vi "GetChildByName.vi"(8 "error in (no error)":errorcluster, 10 "BrowerComponentID(\"\")":string, 11 "reference in":refnum<class "BrowerComponent.lvclass">) -> (0 "error out":errorcluster, 2 "BrowerComponent":refnum<class "BrowerComponent.lvclass">, 3 "reference out":refnum<class "BrowerComponent.lvclass">)   [LabVIEW 2015, in "BrowerComponent.lvclass"]
uses:
  BrowerComponent.lvclass
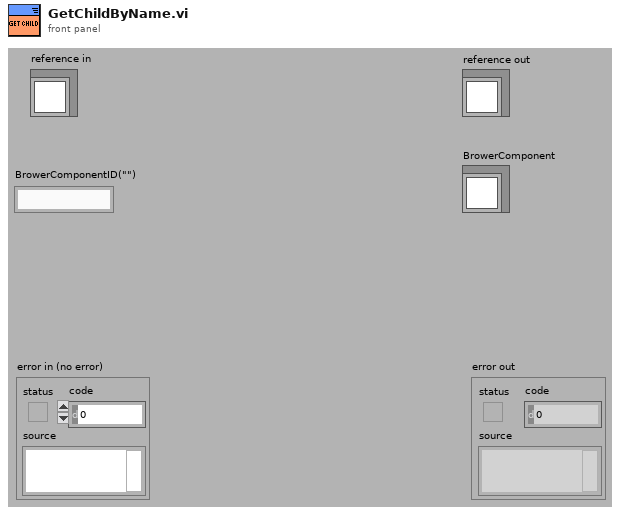
[diagram p1: front panel]
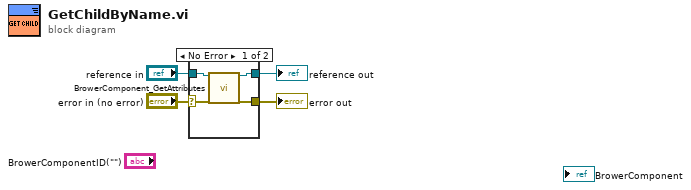
[diagram p0: block diagram]
diagram:
  n1 = case shown="No Error" "error in (no error)" {
    selector: "error in (no error)" -> [w8 w10]
    tunnel: [w7 w10] -> w3
    tunnel: [w5 w9] -> w1
    tunnel: "reference in" -> [w6 w9]
    frame No Error {
      n2 = call "BrowerComponent_GetAttributes.vi"("reference in"=w6, "error in (no error)"=w8) -> ("reference out"=w5:refnum<class "BrowerComponent.lvclass">, "error out"=w7:errorcluster)  [unwired: 14 in, 2 out]
    }
    frame Error {
    }
  }
  "error out" <- w3
  "reference out" <- w1
